vi "Run Bitfile.vi"() -> ()   [LabVIEW 2011]
uses:
  <vilib>/Platform/TimedLoop/XDataNode/timing_clust.ctl
  <vilib>/Platform/TimedLoop/XDataNode/nitl_modes.ctl
  <vilib>/Platform/TimedLoop/XDataNode/wakeup.ctl
  <vilib>/FPGAPlugInAG/sbRIO-9606/niLvFpga_Open_sbRIO-9606.vi
  <vilib>/rvi/interface/common/dynamic/niFpgaDynamicAddResources.vi
  <vilib>/Utility/error.llb/Error Cluster From Error Code.vi
  <vilib>/rvi/errors/niLvFpgaAdjustHostInterfaceError.vi
  <vilib>/FPGAPlugInAG/Dynamic/niLvFpga_Close_Dynamic.vi
  <vilib>/Platform/TimedLoop/XDataNode/XDataNode.xnode
  <vilib>/rvi/interface/nirviOpenFPGA/nirviOpenFPGA.xnode
  natcar/labview/FPGA Bitfiles/natcar_FPGATarget_Top-Level_610FB000.lvbitx
  <vilib>/rvi/interface/nirviReadWriteControl/nirviReadWriteControl.xnode
  <vilib>/rvi/interface/nirviCloseFPGA/nirviCloseFPGA.xnode
  <vilib>/Platform/TimedLoop/XDataNode/XDNodeRunTimeDep.lvlib
  NiFpgaLv.dll
  <vilib>/rvi/interface/Simulation/niFpgaSimulationCallBeginRW.vi
panel:
  out "Raw Sensor Data":T1(graph)
  out "Go Duty":u16
  out "Servo 1e-7s":u32
  out "Line Error Graph":dbl(graph)
  out "Line Error (cm)":dbl
  in  "Steering Kp":dbl min=0.0 max=1000.0 step=1.0
  out "really lost":bool
  out "line found":bool
  out "SC":bool
  out "S5":bool
  out "S4":bool
  out "S3":bool
  out "S2":bool
  out "S1":bool
  out "AI7":u16
  out "AI6":u16
  out "AI5":u16
  out "AI4":u16
  out "AI3":u16
  out "AI2":u16
  out "AI1":u16
  out "AI0":u16
  out "Speed Error":dbl(graph)
  in  "Offset":dbl=22.0 min=0.0 max=30.0 step=0.1
  out "Velocity counts":u32
  out "V [m/s]":dbl
  in  "RUN!":bool
  in  "Stop":bool
  in  "Kff":dbl=6.0 min=0.0 max=10.0 step=0.1
  in  "uBlaze Reset":bool
  in  "Steering ON 1e-7s":u32=15000 min=10240 max=19650 step=100
  in  "Steering":bool
  in  "Throttle":bool
  in  "GO frequency (Hz)":u16=1000 min=10 max=10000 step=10
  in  "GO duty (100*%)":u16 max=100 step=1
  in  "Vdes [m/s]":dbl min=0.0 max=5.0 step=0.1
  in  "Speed Ki":dbl=0.1 min=0.0 max=2.0 step=0.01
  in  "Throttle ON":bool
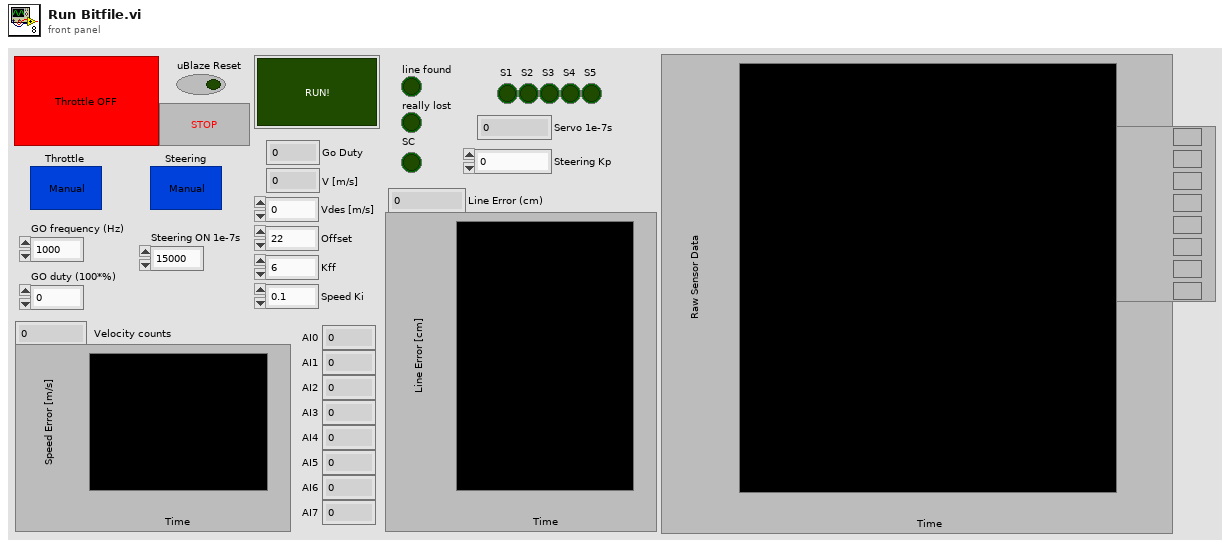
[diagram p1: front panel]
types:
  T1 = cluster{"AI0":u16, "AI1":u16, "AI2":u16, "AI3":u16, "AI4":u16, "AI5":u16, "AI6":u16, "AI7":u16}
  T2 = typedef "XDNodeRunTimeDep.lvlib/timing_clust.ctl" = cluster{"Expected End [f-1]":u64, "Actual End [f-1]":u64, "Finished Late? [f-1]":bool, "Expected End [i-1]":u64, "Actual End [i-1]":u64, "Finished Late? [i-1]":bool, "Expected Start [i]":u64, "Actual Start [i]":u64, "Expected Start [f]":u64, "Actual Start [f]":u64, "Source Name":string, "Structure Name":string, "Period":i64, "Deadline":i64, "Offset":i64, "Start":i64, "Priority":i32, "Timeout":i32, "Mode":T3, "Wakeup Reason":T4, "Error":errorcluster, "Source Type":string, "Secondary Source Type":string, "Global End Time":u64, "Global Start Time":u64, "Frame Duration":u64, "Iteration Duration":u64, "Assigned CPU":i32, "I/O Scan Engine Mode":u32}
  T3 = typedef "XDNodeRunTimeDep.lvlib/nitl_modes.ctl" = enum32{"No Change", "Process missed periods, maintain original phase", "Discard missed periods, maintain original phase", "Process missed periods, ignore original phase", "Discard missed periods, ignore original phase"}
  T4 = typedef "XDNodeRunTimeDep.lvlib/wakeup.ctl" = enum32{"Normal", "Aborted", "Asynchronous wakeup", "Timing source error", "Timed loop error", "Timeout"}
  T5 = cluster{"AI5":u16, "AI6":u16, "AI7":u16, "AI2":u16, "AI1":u16, "AI3":u16, "AI4":u16, "AI0":u16}
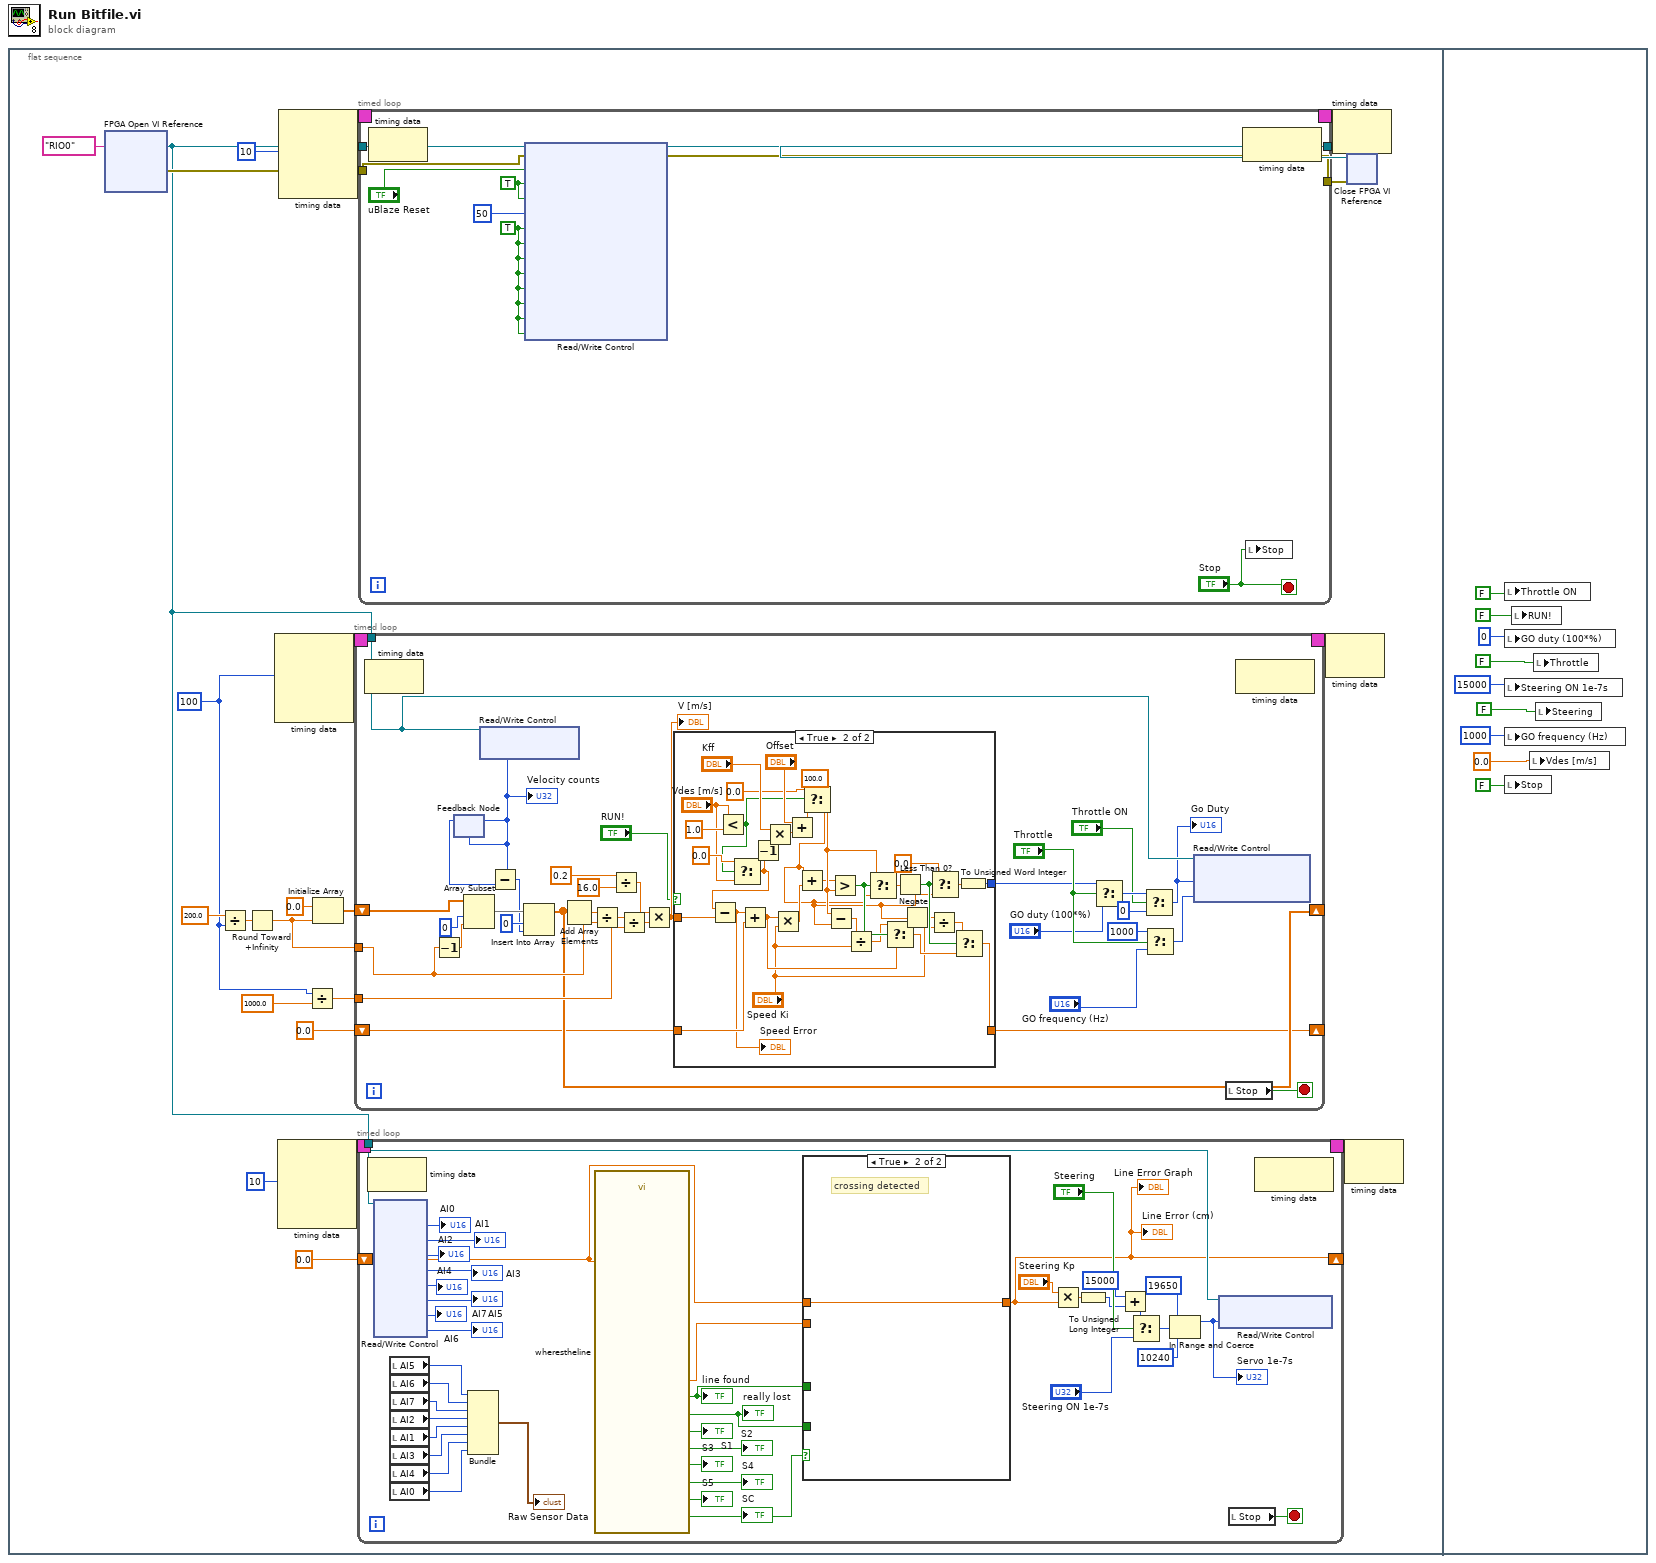
[diagram p0: block diagram]
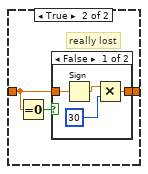
[diagram p4: hidden frame]
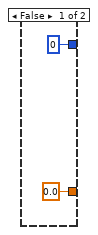
[diagram p6: hidden frame]
diagram:
  n1 = flat-sequence {
    frame #0 {
      w3 = i64 100 ("Period")
      n2 = xnode "FPGA Open VI Reference"("resource name"=tag "RIO0") -> ("FPGA VI Reference Out"=w2:refnum<k20>, "error out"=w16:errorcluster)  [unwired: 1 in]
      n3 = Divide(x=200.0, y=w3) -> (x/y=w10:dbl)
      n4 = Round Toward +Infinity(x=w10) -> (ceil(x): smallest int >= x=w9:dbl)
      n5 = node-c288(w3) -> (w23:T2)  [unwired: 3 in]
      n6 = node-c288(i64 10 ("Period")) -> (w21:T2)  [unwired: 3 in]
      n7 = node-c288(i64 10 ("Period")) -> (w19:T2)  [unwired: 3 in]
      n8 = Divide(x=w3, y=1000.0) -> (x/y=w5:dbl)
      n9 = Initialize Array(0.0 ("element"), w9) -> (w13:dbl[])
      n10 = timed-loop {
        timing: w23 -> [_]
        timing-out: [_] -> w22
        shift-right: [w135] -> _
        shift-left: w13 -> [w134]
        tunnel: w9 -> [w137]
        tunnel: w5 -> [w136]
        shift-right: [w132] -> _
        shift-left: 0.0 -> [w133]
        tunnel: w2 -> [w131]
        stop <- w130 stop-if-true
        n11 = node-c288() -> ()  [unwired: 1 in, 1 out]
        n12 = Decrement(x=w137) -> (x-1=w118:dbl)
        n13 = Array Subset(array=w134, index=0, length=w118) -> (w110:dbl[])
        n14 = xnode "Read/Write Control"("FPGA VI Reference In"=w131) -> ("Velocity counts"=w106:u32)  [unwired: 1 in, 2 out]
        "Velocity counts" <- w106
        n15 = feedback #1(w106) -> (w107:u32)
        n16 = feedback-in #1(w106) -> ()
        n17 = Subtract(x=w106, y=w107) -> (x-y=w109:u32)
        n18 = Insert Into Array(array=w110, index=0, new element=w109) -> (w135:dbl[])
        n19 = Add Array Elements(numeric array=w135) -> (sum=w108:dbl)
        n20 = Divide(x=w108, y=w137) -> (x/y=w116:dbl)
        n21 = Divide(x=0.2, y=16.0) -> (x/y=w112:dbl)
        n22 = Divide(x=w116, y=w136) -> (x/y=w113:dbl)
        n23 = Multiply(x=w112, y=w113) -> (x*y=w111:dbl)
        "V [m/s]" <- w111
        n24 = case shown="True" "RUN!" {
          tunnel: w133 -> [_ w171]
          tunnel: [0.0 w170] -> w132
          tunnel: [u16 0 w169] -> w125
          tunnel: w111 -> [_ w168]
          frame False {
          }
          frame True {
            w162 = 100.0 ("y")
            n25 = Less?(x="Vdes [m/s]", y=1.0) -> (x < y?=w144:bool)
            n26 = Select(t=0.0, s=w144, f="Vdes [m/s]") -> (s? t:f=w145:dbl)
            n27 = Subtract(x=w145, y=w168) -> (x-y=w140:dbl)
            "Speed Error" <- w140
            n28 = Add(x=w140, y=w171) -> (x+y=w155:dbl)
            n29 = Decrement(x=w145) -> (x-1=w146:dbl)
            n30 = Multiply(x="Kff", y=w146) -> (x*y=w149:dbl)
            n31 = Multiply(x=w155, y="Speed Ki") -> (x*y=w167:dbl)
            n32 = Add(x="Offset", y=w149) -> (x+y=w142:dbl)
            n33 = Select(t=0.0, s=w144, f=w142) -> (s? t:f=w141:dbl)
            n34 = Add(x=w141, y=w167) -> (x+y=w158:dbl)
            n35 = Subtract(x=w162, y=w141) -> (x-y=w161:dbl)
            n36 = Greater?(x=w158, y=w162) -> (0:w163:bool)
            n37 = Divide(x=w161, y="Speed Ki") -> (x/y=w160:dbl)
            n38 = Select(t=w162, s=w163, f=w141) -> (s? t:f=w164:dbl)
            n39 = Select(t=w160, s=w163, f=w155) -> (s? t:f=w153:dbl)
            n40 = Less Than 0?(x=w164) -> (x < 0?=w159:bool)
            n41 = Negate(x=w141) -> (-x=w157:dbl)
            n42 = Divide(x=w157, y="Speed Ki") -> (x/y=w156:dbl)
            n43 = Select(t=0.0, s=w159, f=w141) -> (s? t:f=w154:dbl)
            n44 = Select(t=w156, s=w159, f=w153) -> (s? t:f=w170:dbl)
            n45 = To Unsigned Word Integer(number=w154) -> (unsigned 16bit integer=w169:u16)
          }
        }
        n46 = Select(t=w125, s="Throttle", f="GO duty (100*%)") -> (s? t:f=w122:u16)
        n47 = Select(t=w122, s="Throttle ON", f=u16 0 ("t")) -> (s? t:f=w121:u16)
        "Go Duty" <- w121
        n48 = Select(t=u16 1000, s="Throttle", f="GO frequency (Hz)") -> (s? t:f=w124:u16)
        n49 = xnode "Read/Write Control"("FPGA VI Reference In"=w131, "GO duty (100*%)"=w121, "GO frequency (Hz)"=w124) -> ()  [unwired: 1 in, 2 out]
        n50 = local read "Stop"() -> (w130:bool)
        n51 = node-c288() -> ()  [unwired: 1 in, 1 out]
      }
      n52 = timed-loop {
        timing: w21 -> [_]
        timing-out: [_] -> w20
        tunnel: w2 -> [w51]
        shift-right: [w50] -> _
        shift-left: 0.0 -> [w65]
        stop <- w78 stop-if-true
        n53 = node-c288() -> ()  [unwired: 1 in, 1 out]
        n54 = xnode "Read/Write Control"("FPGA VI Reference In"=w51) -> ("AI0"=→"AI0":u16, "AI1"=→"AI1":u16, "AI2"=→"AI2":u16, "AI3"=→"AI3":u16, "AI4"=→"AI4":u16, "AI5"=→"AI5":u16, "AI6"=→"AI6":u16, "AI7"=→"AI7":u16)  [unwired: 1 in, 2 out]
        n55 = local read "AI5"() -> (w47:u16)
        n56 = local read "AI6"() -> (w46:u16)
        n57 = local read "AI7"() -> (w45:u16)
        n58 = local read "AI2"() -> (w44:u16)
        n59 = local read "AI1"() -> (w40:u16)
        n60 = local read "AI3"() -> (w41:u16)
        n61 = local read "AI4"() -> (w42:u16)
        n62 = local read "AI0"() -> (w43:u16)
        n63 = Bundle("AI5"=w47, "AI6"=w46, "AI7"=w45, "AI2"=w44, "AI1"=w40, "AI3"=w41, "AI4"=w42, "AI0"=w43) -> (→"Raw Sensor Data":T5)  [unwired: 1 in]
        n64 = call "wherestheline.vi"("last error"=w65) -> ("SC"=w61:bool, "error"=w64:dbl, "line found"=w66:bool, "really lost"=w62:bool, "S1"=→"S1":bool, "S2"=→"S2":bool, "S3"=→"S3":bool, "S4"=→"S4":bool, "S5"=→"S5":bool)  [unwired: 18 in]
        "SC" <- w61
        "line found" <- w66
        "really lost" <- w62
        n65 = case shown="True" w61 {
          tunnel: w66 -> [w84 _]
          tunnel: w65 -> [w83 w98]
          tunnel: w64 -> [w82 _]
          tunnel: [w81 w98] -> w50
          tunnel: w62 -> [w80 _]
          frame False {
            # "no crossing"
            n66 = case shown="True" w84 {
              tunnel: w83 -> [w86 _]
              tunnel: w82 -> [_ w97]
              tunnel: [w85 w97] -> w81
              tunnel: w80 -> [w87 _]
              frame False {
                # "line not found"
                n67 = case shown="False" w87 {
                  tunnel: [w88 w90] -> w85
                  tunnel: w86 -> [w88 w89]
                  frame False {
                    # "not really lost"
                  }
                  frame True {
                    # "really lost"
                    n68 = Equal To 0?(x=w89) -> (x = 0?=w91:bool)
                    n69 = case shown="False" w91 {
                      tunnel: [w92 w96] -> w90
                      tunnel: w89 -> [w95 w96]
                      frame False {
                        n70 = Sign(1:w95) -> (0:w94:dbl)
                        n71 = Multiply(x=w94, y=u16 30) -> (x*y=w92:dbl)
                      }
                      frame True {
                      }
                    }
                  }
                }
              }
              frame True {
                # "line is found"
              }
            }
          }
          frame True {
            # "crossing detected"
          }
        }
        "Line Error (cm)" <- w50
        "Line Error Graph" <- w50
        n72 = Multiply(x="Steering Kp", y=w50) -> (x*y=w59:dbl)
        n73 = To Unsigned Long Integer(number=w59) -> (unsigned 32bit integer=w57:u32)
        n74 = Add(x=u32 15000, y=w57) -> (x+y=w58:u32)
        n75 = Select(t=w58, s="Steering", f="Steering ON 1e-7s") -> (s? t:f=w55:u32)
        n76 = In Range and Coerce(upper limit=u32 19650, x=w55, lower limit=u32 10240) -> (coerced(x)=w52:u32)  [unwired: 1 out]
        "Servo 1e-7s" <- w52
        n77 = xnode "Read/Write Control"("FPGA VI Reference In"=w51, "Steering ON 1e-7s"=w52) -> ()  [unwired: 1 in, 2 out]
        n78 = local read "Stop"() -> (w78:bool)
        n79 = node-c288() -> ()  [unwired: 1 in, 1 out]
      }
      n80 = timed-loop {
        tunnel: w2 -> [w32]
        tunnel: [w31] -> w17
        tunnel: w16 -> [w29]
        tunnel: [w28] -> w15
        timing: w19 -> [_]
        timing-out: [_] -> w18
        stop <- "Stop" stop-if-true
        w24 = TRUE ("Enable AI0")
        w27 = TRUE ("manual steering")
        n81 = node-c288() -> ()  [unwired: 1 in, 1 out]
        n82 = xnode "Read/Write Control"("FPGA VI Reference In"=w32, "error in"=w29, "uBlaze Reset"="uBlaze Reset", "manual steering"=w27, "manual throttle"=w27, "Steering frequency (Hz)"=u16 50, "Enable AI0"=w24, "Enable AI1"=w24, "Enable AI2"=w24, "Enable AI3"=w24, "Enable AI4"=w24, "Enable AI5"=w24, "Enable AI6"=w24, "Enable AI7"=w24) -> ("FPGA VI Reference Out"=w31:refnum<k20>, "error out"=w28:errorcluster)
        n83 = node-c288() -> ()  [unwired: 1 in, 1 out]
        n84 = local write "Stop"("Stop") -> ()
      }
      n85 = node-c288(w22) -> ()  [unwired: 1 out]
      n86 = node-c288(w18) -> ()  [unwired: 1 out]
      n87 = node-c288(w20) -> ()  [unwired: 1 out]
      n88 = xnode "Close FPGA VI Reference"("FPGA VI Reference In"=w17, "error in"=w15) -> ()  [unwired: 1 out]
    }
    frame #1 {
      n89 = local write "Throttle ON"(FALSE ("Throttle ON")) -> ()
      n90 = local write "GO duty (100*%)"(u16 0 ("GO duty (100*%)")) -> ()
      n91 = local write "Steering ON 1e-7s"(u32 15000 ("Steering ON 1e-7s")) -> ()
      n92 = local write "GO frequency (Hz)"(u16 1000 ("GO frequency (Hz)")) -> ()
      n93 = local write "Stop"(FALSE ("Stop")) -> ()
      n94 = local write "RUN!"(FALSE ("START!")) -> ()
      n95 = local write "Vdes [m/s]"(0.0 ("Desired Speed [m/s]")) -> ()
      n96 = local write "Throttle"(FALSE ("Automatic Throttle")) -> ()
      n97 = local write "Steering"(FALSE ("Automatic Steering")) -> ()
    }
  }
